vi "RunProfile.vi"(8 "error in":errorcluster) -> (0 "error out":errorcluster)   [LabVIEW 2010]
doc: "Use this template to build a VI to use as a subVI."
uses:
  <vilib>/Instr/_visa.llb/VISA Configure Serial Port (Instr).vi
panel:
  in  "Tab":enum32{"UI", "Loading"}(tab)
  in  "Profile":u16(ring)=1 caption="曲线" items=["A", "1"]
  in  "Step":u16=1 caption="步骤"
  in  "Delete":bool
  in  "Run":bool
  in  "Exit":bool
  out "Loading":dbl(slide)=100.0 scale=0.0..100.0
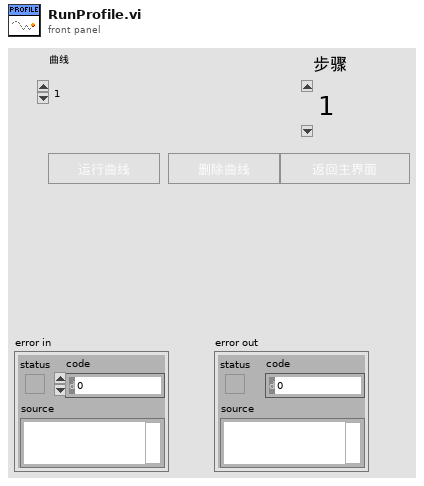
[diagram p1: front panel]
types:
  T1 = enum32{"invalid app kind", "Development System", "Run Time System", "Student Edition", "Embedded LabVIEW", "Evaluation", "Custom"}
  T2 = enum32{"Invalid", "Standard", "Closed", "Hidden", "Minimized", "Maximized"}
  T3 = cluster{"Core":cluster{"Current VI Reference":refnum<vi>, "Close Panel on Exit?":bool}, "Your Boolean data":bool, "Your string data":string}
  T4 = cluster{"Current VI Reference":refnum<vi>, "Close Panel on Exit?":bool}
  T5 = typedef "Path InitPaths__FS.ctl" = cluster{"Ctrller CFG":path, "INI":path, "Profile":path, "EventLog":path, "Data":path}
  T6 = typedef "Controller Configuration__CHC.ctl" = cluster{"Ctrller Type":T7, "Ctrller Name":string, "Ctrller Addr":string, "Server IP":string, "Conn Result":string, "Port":string, "Baud":dbl}
  T7 = typedef "Controller Configuration__Ctrller Type.ctl" = enum16{"F4S/D", "Synergy"}
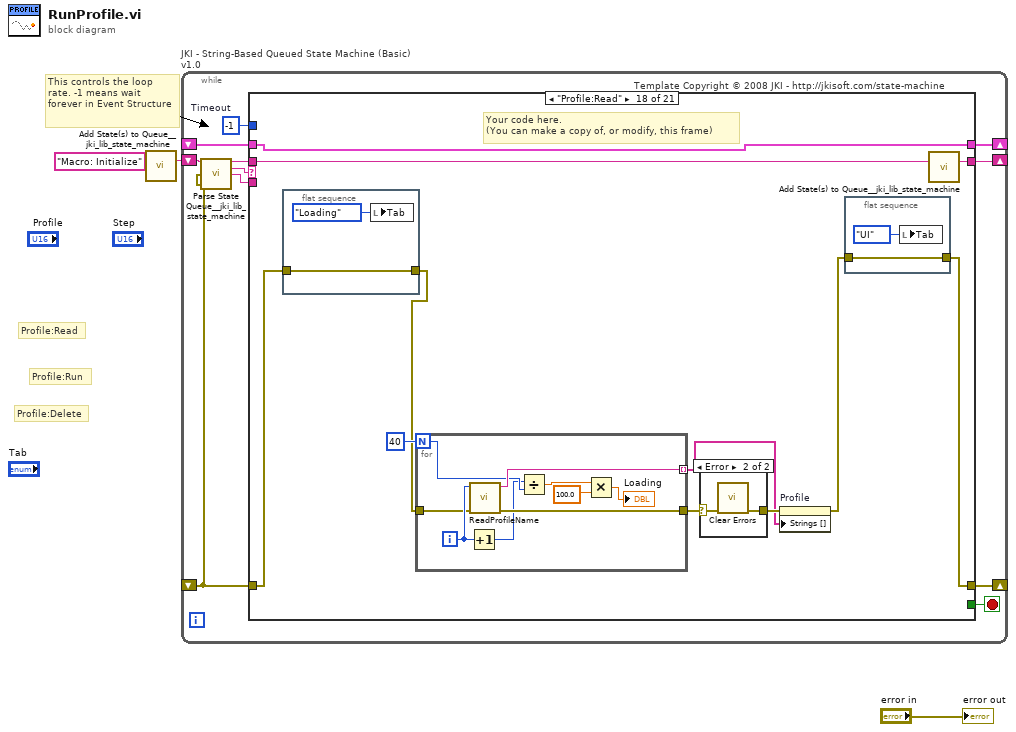
[diagram p0: block diagram]
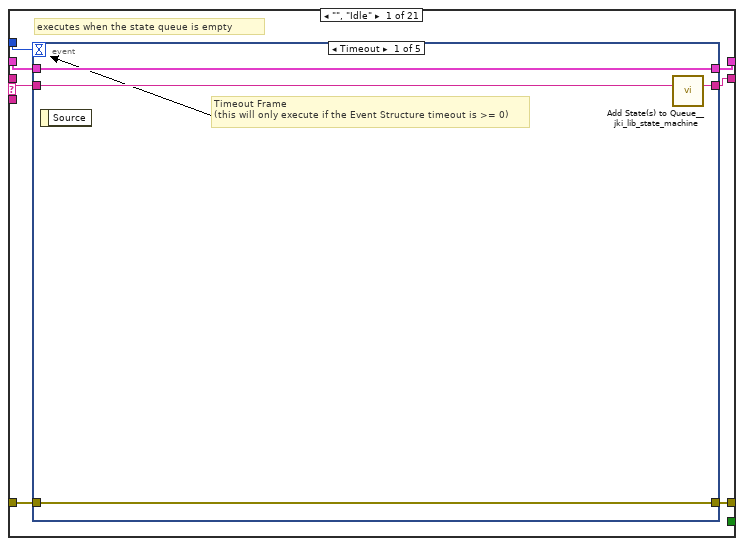
[diagram p2: hidden frame]
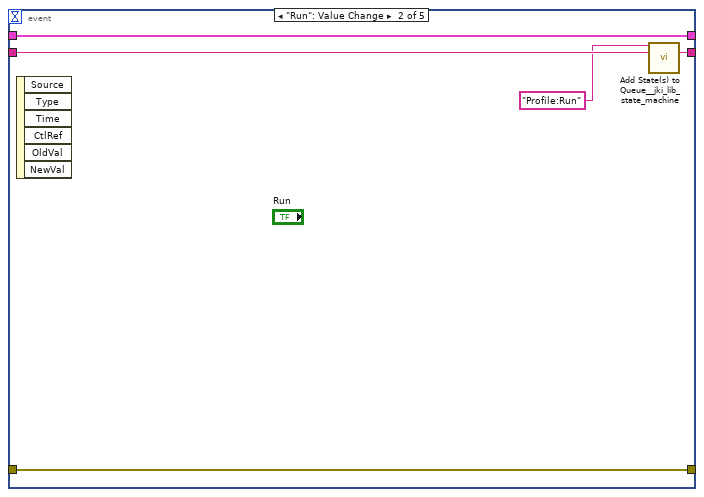
[diagram p3: hidden frame]
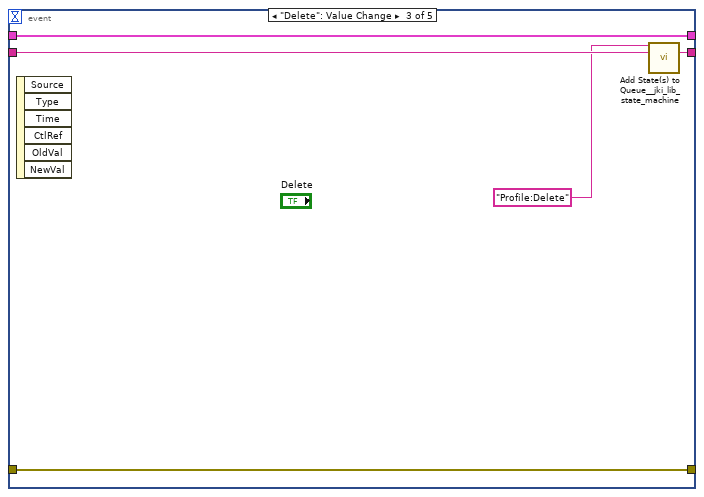
[diagram p4: hidden frame]
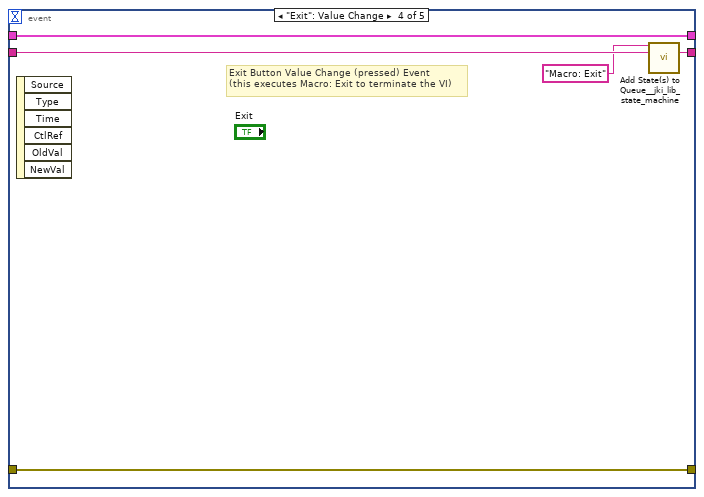
[diagram p5: hidden frame]
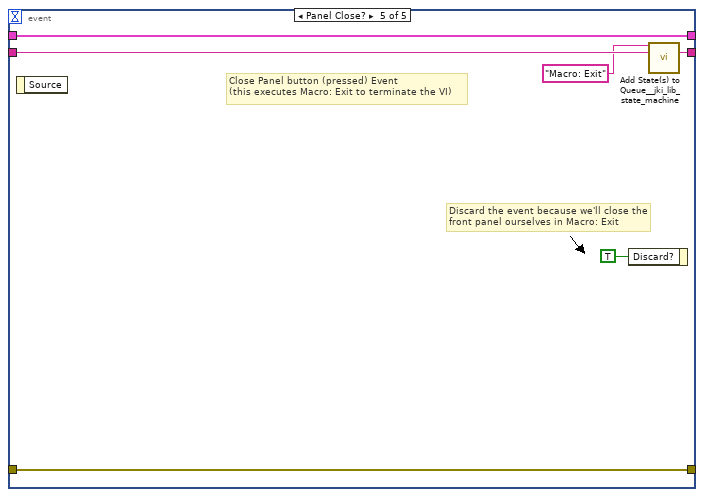
[diagram p6: hidden frame]
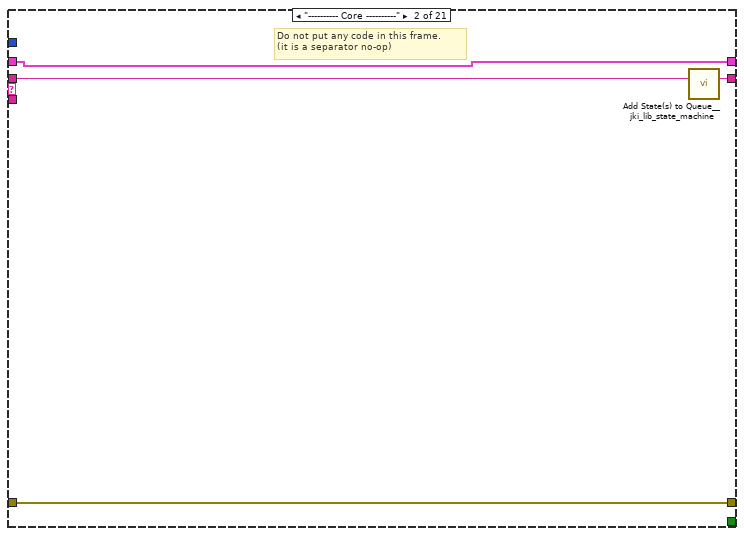
[diagram p7: hidden frame]
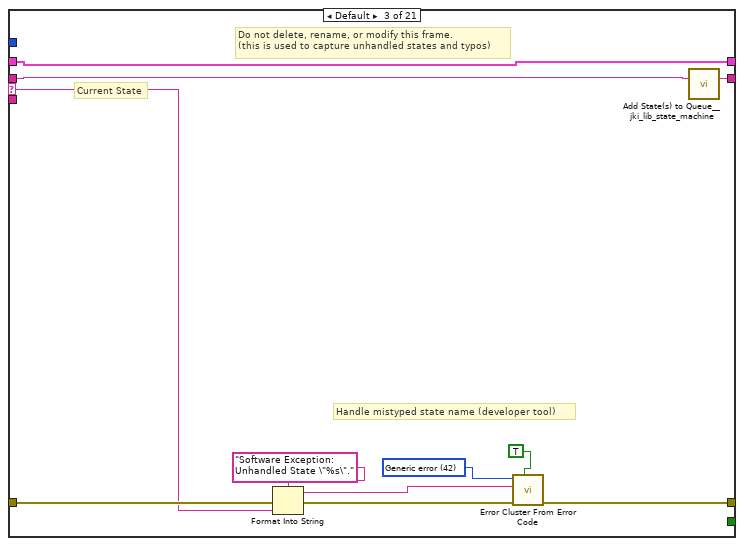
[diagram p8: hidden frame]
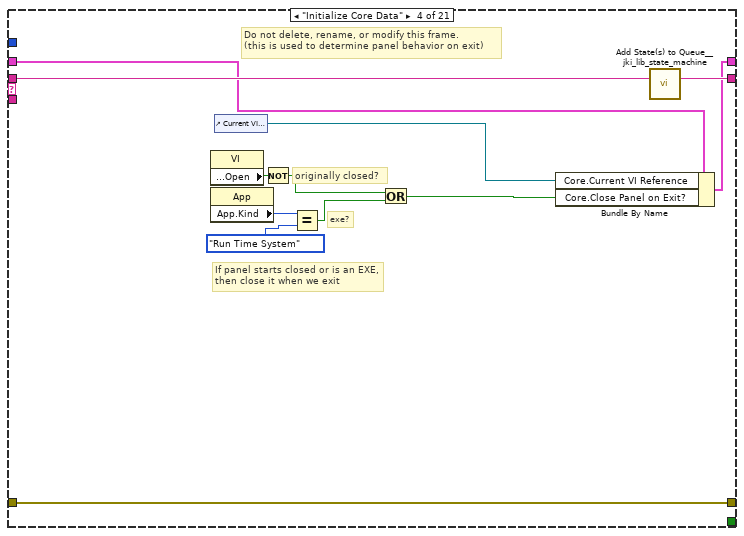
[diagram p9: hidden frame]
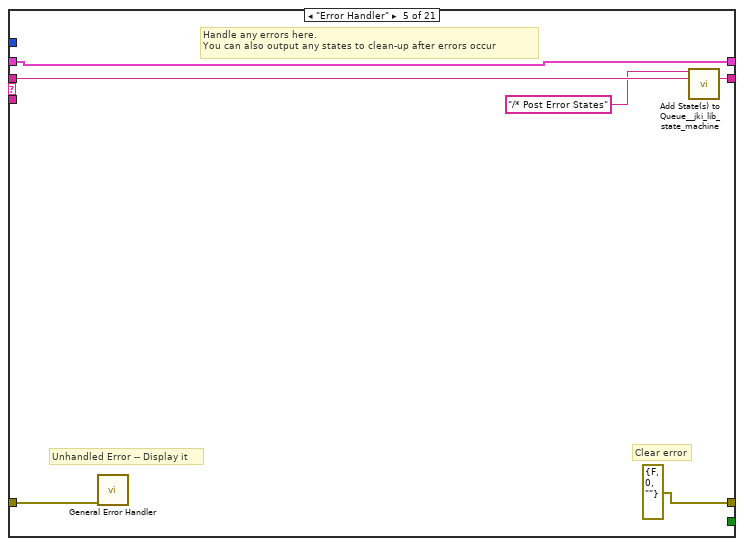
[diagram p10: hidden frame]
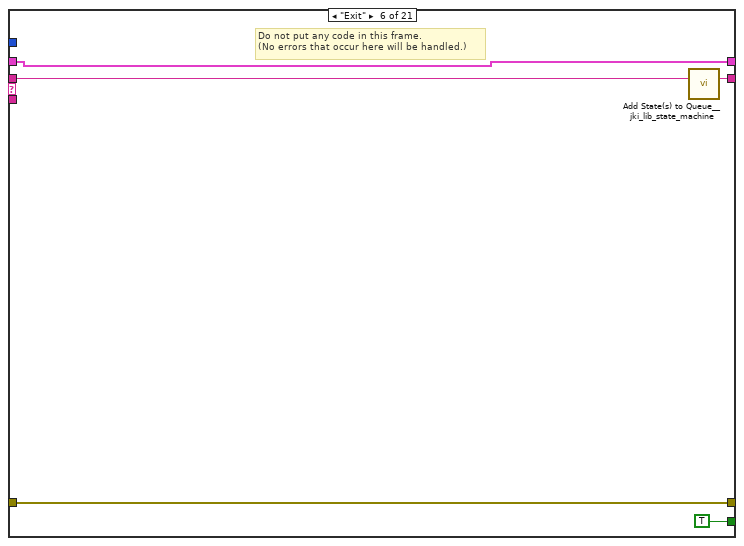
[diagram p11: hidden frame]
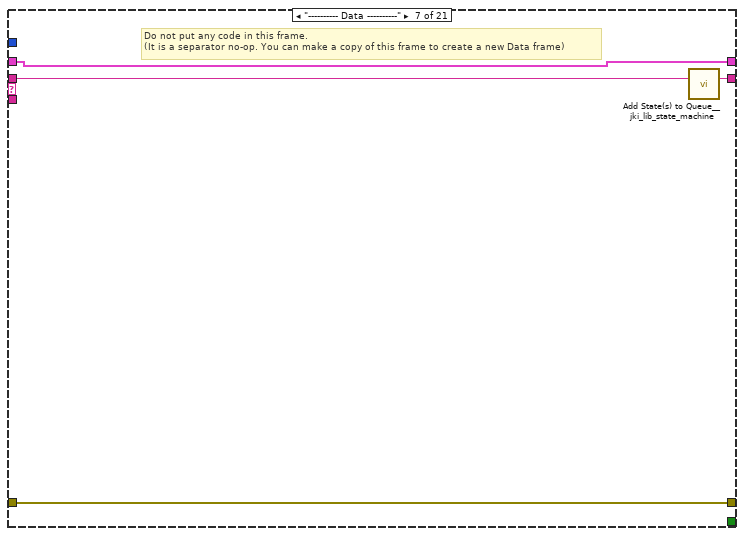
[diagram p12: hidden frame]
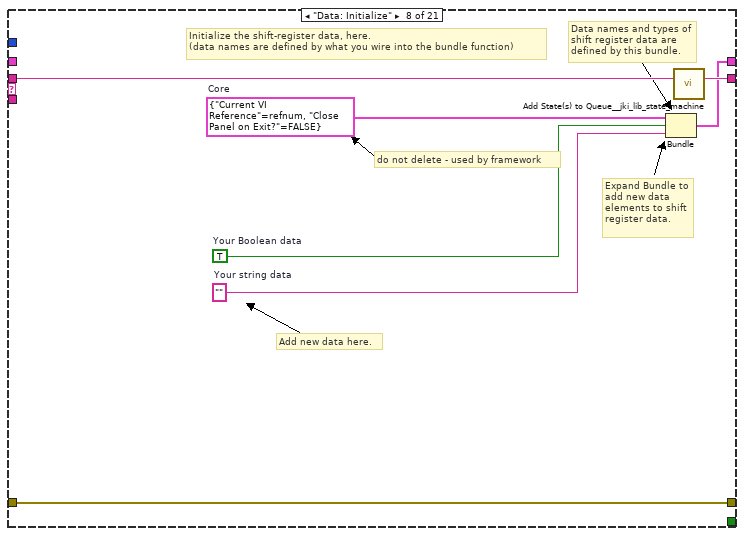
[diagram p13: hidden frame]
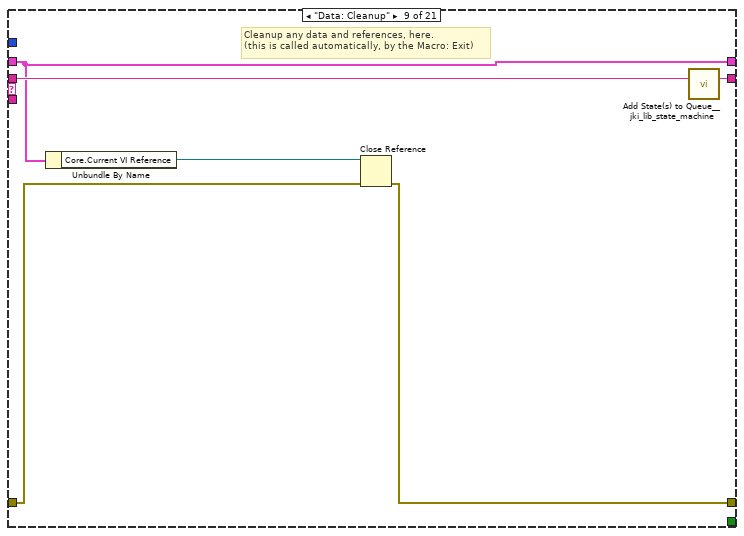
[diagram p14: hidden frame]
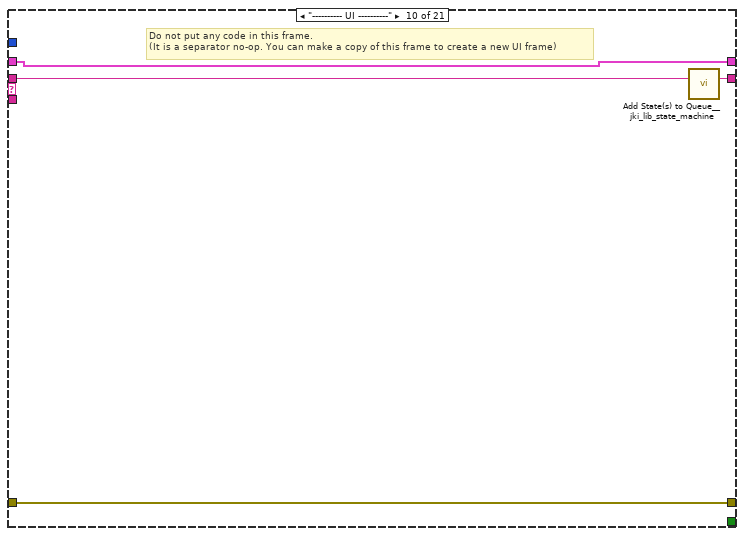
[diagram p15: hidden frame]
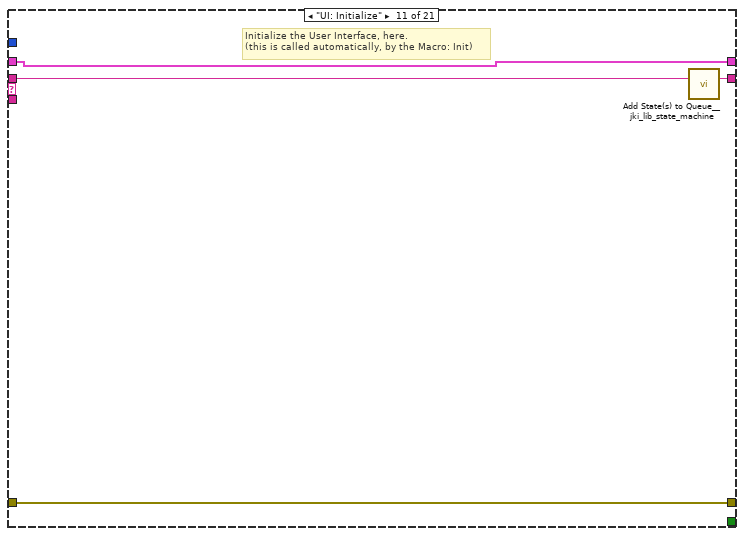
[diagram p16: hidden frame]
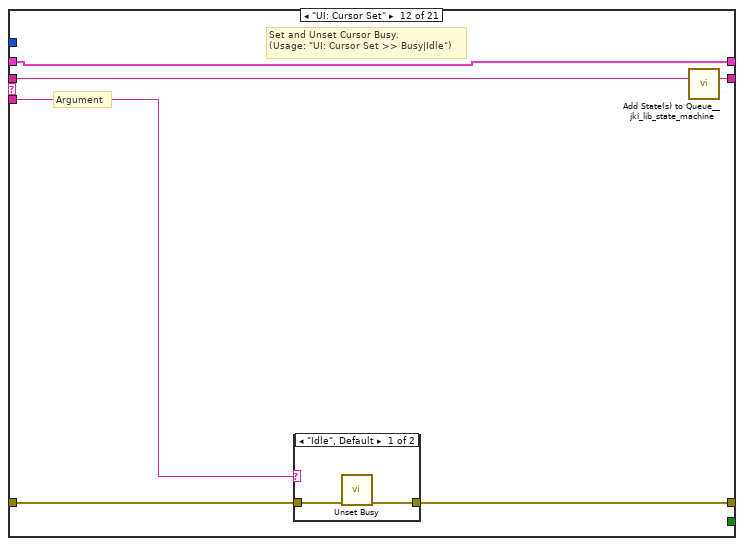
[diagram p17: hidden frame]
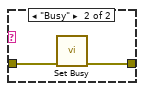
[diagram p18: hidden frame]
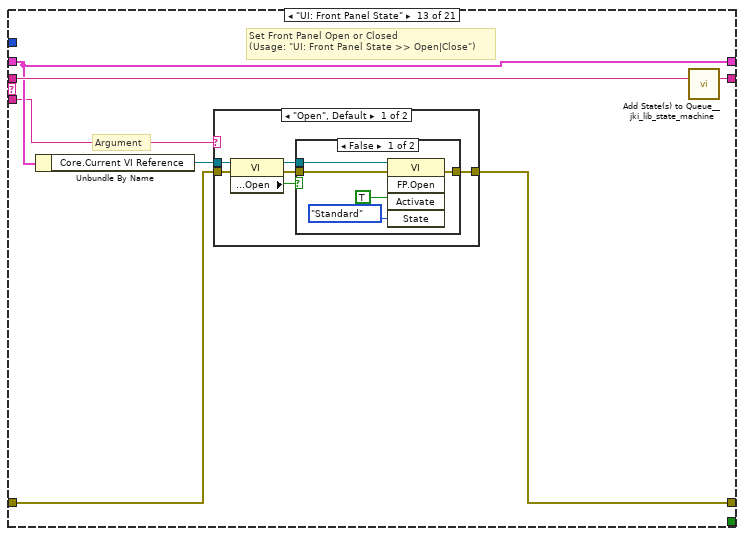
[diagram p19: hidden frame]
diagram:
  # "Profile:Delete"
  # "Profile:Run"
  # "Profile:Read"
  # "This controls the loop rate. -1 means wait forever in Event Structure"
  n1 = call "Add State(s) to Queue__jki_lib_state_machine.vi"("State(s) in (\"\")"="Macro: Initialize") -> ("States Out"=w3:string)  [unwired: 14 in]
  n2 = while "JKI - String-Based Queued State Machine (Basic) v1.0" {
    shift-right: [w7] -> _
    shift-left: _ -> [w6]
    shift-right: [w10] -> _
    shift-left: _ -> [w4]
    shift-right: [w9] -> _
    shift-left: w3 -> [w11]
    stop <- w8 stop-if-true
    w5 = -1  # Timeout
    # "Template Copyright © 2008 JKI - http://jkisoft.com/state-machine"
    n3 = call "Parse State Queue__jki_lib_state_machine.vi"("State Queue"=w11, "Error In (no error)"=w4) -> ("Remaining States"=w13:string, "Current State"=w14:string, "Arguments"=w12:string)  [unwired: 11 in]
    n4 = case shown="\"Profile:Read\"" w14 {
      selector: w14 -> [_ _ w51 _ _ _ _ _ _ _ _ _ _ _ _ _ _ _ _ _ _]
      tunnel: w13 -> [w21 w50 w55 w73 w79 w84 w88 w95 w101 w105 w109 w115 w126 w152 w157 w167 w171 w182 w226 w265 w269]
      tunnel: w12 -> [_ _ _ _ _ _ _ _ _ _ _ w110 w120 _ _ _ _ _ _ _ _]
      tunnel: w6 -> [w19 w47 w53 w64 w76 w82 w85 _ w96 w102 w107 w113 w122 w149 w154 w164 w168 w180 w224 w263 w266]
      tunnel: [w18 w48 w57 w70 errorcluster {"status"=FALSE, "code"=0, "source"=""} ("error out") w81 w86 w92 w97 w103 w106 w111 w123 w150 w155 w165 w169 w177 w200 w239 w267] -> w10
      tunnel: w4 -> [w17 w48 w56 w70 w75 w81 w86 w92 w98 w103 w106 w112 w124 w150 w155 w165 w169 w175 w199 w240 w267]
      tunnel: [w20 w49 w54 w72 w78 w83 w87 w94 w100 w104 w108 w114 w125 w151 w156 w166 w170 w181 w225 w264 w268] -> w9
      tunnel: [_ _ _ _ _ TRUE _ _ _ _ _ _ _ _ _ _ _ _ _ _ _] -> w8
      tunnel: [w16 w47 w53 w71 w76 w82 w85 w93 w96 w102 w107 w113 w122 w149 w154 w164 w168 w180 w224 w263 w266] -> w7
      tunnel: w5 -> [w15 _ _ _ _ _ _ _ _ _ _ _ _ _ _ _ _ _ _ _ _]
      frame "", "Idle" {
        # "executes when the state queue is empty"
        n5 = event shown="[0] Timeout" {
          selector: _ -> [_ _ _ _ _]
          dyn-events: _ -> [_ _ _ _ _]
          timeout: w15 -> [_ _ _ _ _]
          tunnel: w21 -> [w25 w30 w35 w40 w46]
          tunnel: [w24 w29 w34 w39 w45] -> w20
          tunnel: w19 -> [w22 w27 w32 w37 w43]
          tunnel: [w23 w28 w33 w38 w44] -> w18
          tunnel: w17 -> [w23 w28 w33 w38 w44]
          tunnel: [w22 w27 w32 w37 w43] -> w16
          event Timeout {
            # "Timeout Frame\n(this will only execute if the Event Structure timeout is >= 0)"
            n6 = event-data() -> ()  [unwired: 1 in, 1 out]
            n7 = call "Add State(s) to Queue__jki_lib_state_machine.vi"("State(s) in (\"\")"=w25) -> ("States Out"=w24:string)  [unwired: 14 in]
          }
          event "Run": Value Change {
            n8 = event-data() -> ()  [unwired: 1 in, 6 out]
            n9 = call "Add State(s) to Queue__jki_lib_state_machine.vi"("State(s) in Front (\"\")"="Profile:Run" ("State(s) in Front (\"\")"), "State(s) in (\"\")"=w30) -> ("States Out"=w29:string)  [unwired: 13 in]
          }
          event "Delete": Value Change {
            n10 = event-data() -> ()  [unwired: 1 in, 6 out]
            n11 = call "Add State(s) to Queue__jki_lib_state_machine.vi"("State(s) in Front (\"\")"="Profile:Delete" ("State(s) in Front (\"\")"), "State(s) in (\"\")"=w35) -> ("States Out"=w34:string)  [unwired: 13 in]
          }
          event "Exit": Value Change {
            # "Exit Button Value Change (pressed) Event\n(this executes Macro: Exit to terminate the VI)"
            n12 = event-data() -> ()  [unwired: 1 in, 6 out]
            n13 = call "Add State(s) to Queue__jki_lib_state_machine.vi"("State(s) in Front (\"\")"="Macro: Exit", "State(s) in (\"\")"=w40) -> ("States Out"=w39:string)  [unwired: 13 in]
          }
          event Panel Close? {
            # "Discard the event because we'll close the front panel ourselves in Macro: Exit"
            # "Close Panel button (pressed) Event\n(this executes Macro: Exit to terminate the VI)"
            n14 = event-data() -> ()  [unwired: 1 in, 1 out]
            n15 = event-data("Discard?"=TRUE) -> ()  [unwired: 1 in, 1 out]
            n16 = call "Add State(s) to Queue__jki_lib_state_machine.vi"("State(s) in Front (\"\")"="Macro: Exit", "State(s) in (\"\")"=w46) -> ("States Out"=w45:string)  [unwired: 13 in]
          }
        }
      }
      frame "---------- Core ----------" {
        # "Do not put any code in this frame.\n(it is a separator no-op)"
        n17 = call "Add State(s) to Queue__jki_lib_state_machine.vi"("State(s) in (\"\")"=w50) -> ("States Out"=w49:string)  [unwired: 14 in]
      }
      frame Default {
        w60 = 42 items=["No error", "Argument error", "Memory is full", "Out of zone", "End of file", "File already open", "Generic file I/O error", "File not found", "File permission error", "Disk is full", "Duplicate path", "Too many files open", "System feature not enabled", "Resource file not found", "Cannot add resource", "Resource not found", "Image not found", "Image memory error", "Pen does not exist", "Config type invalid", "Config token not found", "Config parse error", "Config memory error", "Bad external code format", "Bad external code offset", "External code not present", "Null window", "Destroy window error", "Null menu", "Print aborted", "Bad print record", "Print driver error", "Windows error during printing", "Memory error during printing", "Print dialog error", "Generic print error", "Invalid device refnum", "Device not found", "Device parameter error", "Device unit error", "Cannot open device", "Device call aborted", "Generic error", "Cancelled by user", "Object ID too low", "Object ID too high", "Object not in heap", "Unknown heap", "Unknown object (invalid DefProc)", "Unknown object (DefProc not in table)", "Message out of range", "Invalid (null) method", "Unknown message", "Manager call not supported", "Bad address", "Network operation in progress", "Network operation timed out", "Connection is busy", "Network attribute not supported", "Network error", "Address in use", "System out of memory", "Connection aborted", "Connection refused", "Not connected", "Already connected", "Connection closed", "Initialization error (interapplication manager)", "Bad occurrence", "Wait on unbound occurrence handler", "Occurrence queue overflow", "Datalog type conflict", "Unused", "Unrecognized type (interapplication manager)", "Memory corrupt", "Failed to make temporary DLL", "Old CIN version", "Drag socket not found", "Failed to load drop-object", "Failed to register OLE object", "Failed to release OLE object", "Format specifier type mismatch", "Unknown format specifier", "Too few format specifiers", "Too many format specifiers", "Scan failed", "Newer CIN version", "Error converting to variant", "Runtime menu error", "Password tampered", "Variant attribute not found", "Incompatible variant data type", "Event data is not available", "Event Store is not present", "Occurrence is not found", "Event Queue is not created", "Event info is not available", "Refnum passed is NULL", "Error retrieving Class GUID", "Error retrieving CoClass GUID", "Error retrieving TypeLib GUID.", "Bad built application magic bytes.", "Specific driver is different from the specific driver associated with the Logical Name.", "There is no session opened to the class driver.", "Max Error", "MAX - Error with config objects", "MAX - Error loading configuration", "MAX - Group not supported"]
        # "Current State"
        # "Do not delete, rename, or modify this frame.\n(this is used to capture unhandled states and typos)"
        # "Handle mistyped state name (developer tool)"
        n18 = Format Into String(format string="Software Exception: Unhandled State \"%s\"." ("message"), error in=w56, w51) -> (resulting string=w59:string, error out=w58:errorcluster)  [unwired: 1 in]
        n19 = call <vilib>:"Error Cluster From Error Code.vi"("show call chain? (False)"=TRUE, "error in (no error)"=w58, "error message (\"\")"=w59, "error code (0)"=w60) -> ("error out"=w57:errorcluster)  [unwired: 5 in]
        n20 = call "Add State(s) to Queue__jki_lib_state_machine.vi"("State(s) in (\"\")"=w55) -> ("States Out"=w54:string)  [unwired: 14 in]
      }
      frame "Initialize Core Data" {
        # "Do not delete, rename, or modify this frame.\n(this is used to determine panel behavior on exit)"
        # "originally closed?"
        # "exe?"
        # "If panel starts closed or is an EXE, then close it when we exit"
        n21 = property class="VI"() -> ("Front Panel.Open"=w69:bool)  [unwired: 2 in, 2 out]
        n22 = property class="App"() -> ("App.Kind"=w68:T1)  [unwired: 2 in, 2 out]
        n23 = control-ref of="Current VI Reference"() -> (w62:refnum<vi>)
        n24 = Not(x=w69) -> (.not. x?=w66:bool)
        n25 = Equal?(x=w68, y=T1."Run Time System" ("Application:Kind")) -> (x = y?=w65:bool)
        n26 = Or(x=w66, y=w65) -> (x .or. y?=w63:bool)
        n27 = Bundle By Name(cluster=w64, "Core.Current VI Reference"=w62, "Core.Close Panel on Exit?"=w63) -> (w71:T3)
        n28 = call "Add State(s) to Queue__jki_lib_state_machine.vi"("State(s) in (\"\")"=w73) -> ("States Out"=w72:string)  [unwired: 14 in]
      }
      frame "Error Handler" {
        # "Unhandled Error -- Display it"
        # "Handle any errors here.\nYou can also output any states to clean-up after errors occur"
        # "Clear error"
        n29 = call <vilib>:"General Error Handler.vi"("error in (no error)"=w75) -> ()  [unwired: 10 in, 5 out]
        n30 = call "Add State(s) to Queue__jki_lib_state_machine.vi"("State(s) in Front (\"\")"="/* Post Error States", "State(s) in (\"\")"=w79) -> ("States Out"=w78:string)  [unwired: 13 in]
      }
      frame "Exit" {
        # "Do not put any code in this frame.\n(No errors that occur here will be handled.)"
        n31 = call "Add State(s) to Queue__jki_lib_state_machine.vi"("State(s) in (\"\")"=w84) -> ("States Out"=w83:string)  [unwired: 14 in]
      }
      frame "---------- Data ----------" {
        # "Do not put any code in this frame.\n(It is a separator no-op. You can make a copy of this frame to create a new Data frame)"
        n32 = call "Add State(s) to Queue__jki_lib_state_machine.vi"("State(s) in (\"\")"=w88) -> ("States Out"=w87:string)  [unwired: 14 in]
      }
      frame "Data: Initialize" {
        w89 = T4 {"Current VI Reference"=refnum, "Close Panel on Exit?"=FALSE}  # Core
        w91 = TRUE  # Your Boolean data
        w90 = ""  # Your string data
        # "do not delete - used by framework"
        # "Expand Bundle to add new data elements to shift register data."
        # "Add new data here."
        # "Data names and types of shift register data are defined by this bundle."
        # "Initialize the shift-register data, here.\n(data names are defined by what you wire into the bundle function)"
        n33 = Bundle("Core"=w89, "Your Boolean data"=w91, "Your string data"=w90) -> (w93:T3)  [unwired: 1 in]
        n34 = call "Add State(s) to Queue__jki_lib_state_machine.vi"("State(s) in (\"\")"=w95) -> ("States Out"=w94:string)  [unwired: 14 in]
      }
      frame "Data: Cleanup" {
        # "Cleanup any data and references, here.\n(this is called automatically, by the Macro: Exit)"
        n35 = Unbundle By Name(w96) -> ("Core.Current VI Reference"=w99:refnum<vi>)
        n36 = Close Reference(reference=w99, error in (no error)=w98) -> (error out=w97:errorcluster)
        n37 = call "Add State(s) to Queue__jki_lib_state_machine.vi"("State(s) in (\"\")"=w101) -> ("States Out"=w100:string)  [unwired: 14 in]
      }
      frame "---------- UI ----------" {
        # "Do not put any code in this frame.\n(It is a separator no-op. You can make a copy of this frame to create a new UI frame)"
        n38 = call "Add State(s) to Queue__jki_lib_state_machine.vi"("State(s) in (\"\")"=w105) -> ("States Out"=w104:string)  [unwired: 14 in]
      }
      frame "UI: Initialize" {
        # "Initialize the User Interface, here.\n(this is called automatically, by the Macro: Init)"
        n39 = call "Add State(s) to Queue__jki_lib_state_machine.vi"("State(s) in (\"\")"=w109) -> ("States Out"=w108:string)  [unwired: 14 in]
      }
      frame "UI: Cursor Set" {
        # "Argument"
        # "Set and Unset Cursor Busy.\n(Usage: \"UI: Cursor Set >> Busy|Idle\")"
        n40 = case shown="\"Idle\", Default" w110 {
          tunnel: w112 -> [w117 w119]
          tunnel: [w116 w118] -> w111
          frame "Idle", Default {
            n41 = call <vilib>:"Unset Busy.vi"("error in (no error)"=w117) -> ("error out"=w116:errorcluster)  [unwired: 10 in]
          }
          frame "Busy" {
            n42 = call <vilib>:"Set Busy.vi"("error in (no error)"=w119) -> ("error out"=w118:errorcluster)  [unwired: 9 in, 1 out]
          }
        }
        n43 = call "Add State(s) to Queue__jki_lib_state_machine.vi"("State(s) in (\"\")"=w115) -> ("States Out"=w114:string)  [unwired: 14 in]
      }
      frame "UI: Front Panel State" {
        # "Argument"
        # "Set Front Panel Open or Closed\n(Usage: \"UI: Front Panel State >> Open|Close\")"
        n44 = Unbundle By Name(w122) -> ("Core.Current VI Reference"=w121:refnum<vi>)
        n45 = case shown="\"Open\", Default" w120 {
          tunnel: w124 -> [w130 w143]
          tunnel: [w132 w144] -> w123
          tunnel: w121 -> [w131 w141]
          frame "Open", Default {
            n46 = property class="VI"(reference=w131, error in=w130) -> (reference out=w128:refnum<vi>, error out=w129:errorcluster, "Front Panel.Open"=w127:bool)
            n47 = case shown="False" w127 {
              tunnel: [w135 w138] -> w132
              tunnel: w129 -> [w134 w138]
              tunnel: w128 -> [w133 _]
              frame False {
                n48 = invoke class="VI" method="FP.Open"(reference=w133, error in=w134, "Activate"=TRUE, "State"=T2."Standard") -> (error out=w135:errorcluster)  [unwired: 1 in, 4 out]
              }
              frame True {
              }
            }
          }
          frame "Close" {
            n49 = property class="VI"(reference=w141, error in=w143) -> (reference out=w140:refnum<vi>, error out=w142:errorcluster, "Front Panel.Open"=w139:bool)
            n50 = case shown="True" w139 {
              tunnel: [w145 w148] -> w144
              tunnel: w142 -> [w145 w147]
              tunnel: w140 -> [_ w146]
              frame False {
              }
              frame True {
                n51 = invoke class="VI" method="FP.Close"(reference=w146, error in=w147) -> (error out=w148:errorcluster)  [unwired: 1 in, 2 out]
              }
            }
          }
        }
        n52 = call "Add State(s) to Queue__jki_lib_state_machine.vi"("State(s) in (\"\")"=w126) -> ("States Out"=w125:string)  [unwired: 14 in]
      }
      frame "---------- Macro ----------" {
        # "Do not put any code in this frame.\n(It is a separator no-op. You can make a copy of this frame to create a new Macro frame)"
        n53 = call "Add State(s) to Queue__jki_lib_state_machine.vi"("State(s) in (\"\")"=w152) -> ("States Out"=w151:string)  [unwired: 14 in]
      }
      frame "Macro: Initialize" {
        w153 = "Data: Initialize\nInitialize Core Data\nUI: Initialize\nUI: Front Panel State >> Open\nProfile:Read"  # Data: Initialize Initialize Core Data UI: Initialize UI: Front Panel State >> Open Profile:Read
        # "Initialization Macro\n(This is called once, when the VI starts)"
        n54 = call "Add State(s) to Queue__jki_lib_state_machine.vi"("State(s) in Front (\"\")"=w153, "State(s) in (\"\")"=w157) -> ("States Out"=w156:string)  [unwired: 13 in]
      }
      frame "Macro: Exit" {
        # "Exit Macro\n(This is called once, when the VI exits)"
        n55 = Unbundle By Name(w164) -> ("Core.Close Panel on Exit?"=w163:bool)
        n56 = Select(t="UI: Front Panel State >> Close", s=w163, f="") -> (s? t:f=w160:string)
        n57 = call "Add State(s) to Queue__jki_lib_state_machine.vi"("State(s) in (\"\")"=w160, "State(s) at Back (\"\")"="Data: Cleanup\nExit") -> ("States Out"=w158:string)  [unwired: 13 in]
        n58 = call "Add State(s) to Queue__jki_lib_state_machine.vi"("State(s) in Front (\"\")"=w158, "State(s) in (\"\")"=w167) -> ("States Out"=w166:string)  [unwired: 13 in]
      }
      frame "---------- New Category ----------" {
        # "Template Separator\n(You can make a copy of, or modify, this frame)"
        n59 = call "Add State(s) to Queue__jki_lib_state_machine.vi"("State(s) in (\"\")"=w171) -> ("States Out"=w170:string)  [unwired: 14 in]
      }
      frame "Profile:Read" {
        # "Your code here.\n(You can make a copy of, or modify, this frame)"
        n60 = flat-sequence {
          tunnel: [w183] -> w176
          tunnel: w175 -> [w183]
          frame #0 {
            n61 = local write "Tab"(enum32{"UI", "Loading"}."Loading" ("Tab")) -> ()
          }
        }
        n62 = for {
          N: 40 -> [w192]
          tunnel: [w195] -> w173 mode=indexing
          tunnel: [w194] -> w178
          tunnel: w176 -> [w187]
          i -> [w193]
          n63 = Increment(x=w193) -> (x+1=w188:i32)
          n64 = call "ReadProfileName.vi"("error in (no error)"=w187, "ProfileNumber(from 0)"=w193) -> ("error out"=w194:errorcluster, "Profile Names"=w195:string)  [unwired: 8 in]
          n65 = Divide(x=w188, y=w192) -> (x/y=w191:dbl)
          n66 = Multiply(x=w191, y=100.0) -> (x*y=→"Loading":dbl)
        }
        n67 = case shown="Error" w178 {
          selector: w178 -> [w196 w198]
          tunnel: [w196 w197] -> w174
          frame No Error {
          }
          frame Error {
            n68 = call <vilib>:"Clear Errors.vi"("error in (no error)"=w198) -> ("error out"=w197:errorcluster)  [unwired: 6 in]
          }
        }
        n69 = property on="Profile" class="Ring (strict)"(error in=w174, "Strings []"=w173) -> (error out=w172:errorcluster)  [unwired: 1 in, 1 out]
        n70 = flat-sequence {
          tunnel: [w185] -> w177
          tunnel: w172 -> [w185]
          frame #0 {
            n71 = local write "Tab"(enum32{"UI", "Loading"}."UI" ("Tab")) -> ()
          }
        }
        n72 = call "Add State(s) to Queue__jki_lib_state_machine.vi"("State(s) in (\"\")"=w182) -> ("States Out"=w181:string)  [unwired: 14 in]
      }
      frame "Profile:Run" {
        w203 = u16 3 items=["Create Profile", "Delete Current Profile", "Delete Step", "Start Profile", "Delete All Profiles", "Rename Profile"]  # Action (0: Create Profile)
        # "Your code here.\n(You can make a copy of, or modify, this frame)"
        n73 = flat-sequence {
          tunnel: [w227] -> _
          tunnel: w199 -> [w227]
          frame #0 {
            n74 = local write "Tab"(enum32{"UI", "Loading"}."Loading" ("Tab")) -> ()
          }
        }
        n75 = call "File System Paths__FS.vi"("error in (no error)"=w199) -> ("error out"=w211:errorcluster, "FilePaths"=w205:T5)  [unwired: 8 in, 1 out]
        n76 = for {
          N: 40 -> [w233]
          tunnel: w199 -> [_]
          i -> [w234]
          n77 = Increment(x=w234) -> (x+1=w237:i32)
          n78 = Wait (ms)(milliseconds to wait=u32 10) -> ()  [unwired: 1 out]
          n79 = Divide(x=w237, y=w233) -> (x/y=w235:dbl)
          n80 = Multiply(x=w235, y=100.0) -> (x*y=w231:dbl)
          n81 = local write "Loading"(w231) -> ()
        }
        n82 = Unbundle By Name(w205) -> ("Ctrller CFG"=w204:path)
        n83 = call "Ctrller Cfg Read__FS.vi"("error in (no error)"=w211, "Path In"=w204) -> ("error out"=w212:errorcluster, "Ctrllers"=w206:T6[])  [unwired: 7 in, 1 out]
        n84 = Index Array(array=w206, index=0) -> (element=w208:T6)
        n85 = local read "Profile"() -> (w222:u16)
        n86 = Unbundle By Name(w208) -> ("Ctrller Addr"=w209:string, "Port"=w213:string, "Baud"=w210:dbl)  [unwired: 1 out]
        n87 = Increment(x=w222) -> (x+1=w223:u16)
        n88 = local read "Step"() -> (w221:u16)
        n89 = To Long Integer(number=w210) -> (32bit integer=w217:i32)
        n90 = Decimal String To Number(string=w209) -> (number=w214:i32)  [unwired: 2 in, 1 out]
        n91 = call-poly "VISA Configure Serial Port"("VISA resource name"=w213, "timeout (10sec)"=u32 100, "baud rate (9600)"=w217, "error in (no error)"=w212) -> ("VISA resource name out"=w219:refnum<visa-resource-name>, "error out"=w215:errorcluster)  [unwired: 10 in]
        n92 = call "Configure Profile.vi"("VISA resource name"=w219, "Unit Address (1)"=w214, "Action (0: Create Profile)"=w203, "Profile Number (1)"=w223, "Step (1)"=w221, "error in (no error)"=w215) -> ("VISA resource name out"=w218:refnum<visa-resource-name>, "error out"=w216:errorcluster)  [unwired: 8 in]
        n93 = flat-sequence {
          tunnel: [w229] -> _
          tunnel: w200 -> [w229]
          frame #0 {
            n94 = local write "Tab"(enum32{"UI", "Loading"}."UI" ("Tab")) -> ()
          }
        }
        n95 = call <vilib>:"Clear Errors.vi"("error in (no error)"=w216) -> ("error out"=w202:errorcluster)  [unwired: 6 in]
        n96 = VISA Close(VISA resource name=w218, error in (no error)=w202) -> (error out=w200:errorcluster)
        n97 = call "Add State(s) to Queue__jki_lib_state_machine.vi"("State(s) in (\"\")"=w226) -> ("States Out"=w225:string)  [unwired: 14 in]
      }
      frame "Profile:Delete" {
        w242 = u16 1 items=["Create Profile", "Delete Current Profile", "Delete Step", "Start Profile", "Delete All Profiles", "Rename Profile"]  # Action (0: Create Profile)
        # "Your code here.\n(You can make a copy of, or modify, this frame)"
        n98 = call "File System Paths__FS.vi"("error in (no error)"=w240) -> ("error out"=w250:errorcluster, "FilePaths"=w244:T5)  [unwired: 8 in, 1 out]
        n99 = Unbundle By Name(w244) -> ("Ctrller CFG"=w243:path)
        n100 = call "Ctrller Cfg Read__FS.vi"("error in (no error)"=w250, "Path In"=w243) -> ("error out"=w251:errorcluster, "Ctrllers"=w245:T6[])  [unwired: 7 in, 1 out]
        n101 = Index Array(array=w245, index=0) -> (element=w247:T6)
        n102 = local read "Profile"() -> (w261:u16)
        n103 = Unbundle By Name(w247) -> ("Ctrller Addr"=w248:string, "Port"=w252:string, "Baud"=w249:dbl)  [unwired: 1 out]
        n104 = Increment(x=w261) -> (x+1=w262:u16)
        n105 = local read "Step"() -> (w260:u16)
        n106 = To Long Integer(number=w249) -> (32bit integer=w256:i32)
        n107 = Decimal String To Number(string=w248) -> (number=w253:i32)  [unwired: 2 in, 1 out]
        n108 = call-poly "VISA Configure Serial Port"("VISA resource name"=w252, "timeout (10sec)"=u32 100, "baud rate (9600)"=w256, "error in (no error)"=w251) -> ("VISA resource name out"=w258:refnum<visa-resource-name>, "error out"=w254:errorcluster)  [unwired: 10 in]
        n109 = call "Configure Profile.vi"("VISA resource name"=w258, "Unit Address (1)"=w253, "Action (0: Create Profile)"=w242, "Profile Number (1)"=w262, "Step (1)"=w260, "error in (no error)"=w254) -> ("VISA resource name out"=w257:refnum<visa-resource-name>, "error out"=w255:errorcluster)  [unwired: 8 in]
        n110 = call <vilib>:"Clear Errors.vi"("error in (no error)"=w255) -> ("error out"=w241:errorcluster)  [unwired: 6 in]
        n111 = VISA Close(VISA resource name=w257, error in (no error)=w241) -> (error out=w239:errorcluster)
        n112 = call "Add State(s) to Queue__jki_lib_state_machine.vi"("State(s) in Front (\"\")"="Profile:Read" ("State(s) in Front (\"\")"), "State(s) in (\"\")"=w265) -> ("States Out"=w264:string)  [unwired: 13 in]
      }
      frame "New Category: 2" {
        # "Your code here.\n(You can make a copy of, or modify, this frame)"
        n113 = call "Add State(s) to Queue__jki_lib_state_machine.vi"("State(s) in (\"\")"=w269) -> ("States Out"=w268:string)  [unwired: 14 in]
      }
    }
  }
  "error out" <- "error in"
